vi "First.vi"(7 "Address":string, 8 "Error In":errorcluster) -> (0 "Error Out":errorcluster)   [LabVIEW 2018, in "Tests.lvlib" / "Known Hosts.lvlib"]
uses:
  Known Hosts.lvlib
  src/Toolkit/API/Known Hosts/API/Typedefs/Get Results.ctl
  <vilib>/Utility/error.llb/Clear Errors.vi
  <vilib>/Utility/file.llb/Is Path and Not Empty.vi
  <vilib>/Utility/sysdir.llb/Get System Directory.vi
  src/Toolkit/API/Known Host/Support/Create from Known Hosts.vi
  src/Toolkit/API/Known Host/Support/Destroy to Known Hosts.vi
  <vilib>/addons/_JKI Toolkits/Caraya/classes/Test/Test.lvclass
  <vilib>/addons/_JKI Toolkits/Caraya/classes/Assert/Assert.lvclass
  src/Toolkit/API/Known Hosts/Known Hosts.lvclass
  Tests.lvlib
  src/Toolkit/API/Session/Session.lvclass
  src/Toolkit/API/Known Host/Known Host.lvclass
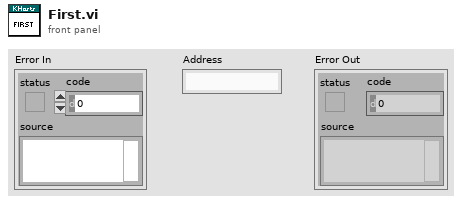
[diagram p1: front panel]
types:
  T1 = typedef "Toolkit.lvlib/Known Hosts.lvclass/Get Results.ctl" = enum32{"Success", "End of Hosts"}
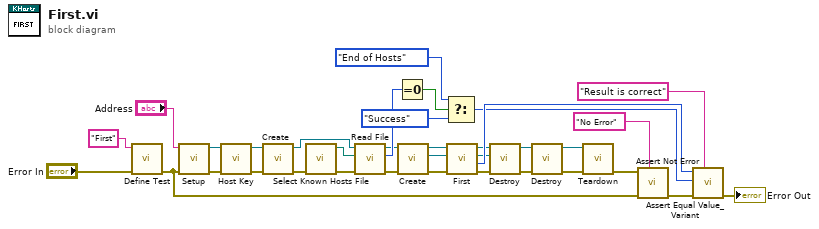
[diagram p0: block diagram]
diagram:
  n1 = call <vilib>:"Define Test.vi"("error in (no error)"="Error In", "Label (VI Title)"="First") -> ("error out"=w22:errorcluster)  [unwired: 9 in]
  n2 = call "Setup.vi"("Error In"=w22, "Address In"="Address") -> ("Error Out"=w23:errorcluster, "Sesssion"=w24:refnum<class "Session.lvclass">)  [unwired: 7 in, 1 out]
  n3 = call "Host Key.vi"("Error In"=w23, "Session In"=w24) -> ("Error Out"=w25:errorcluster, "Sesssion Out"=w20:refnum<class "Session.lvclass">)  [unwired: 6 in, 2 out]
  n4 = call "Create.vi"("Error In"=w25, "Session"=w20) -> ("Error Out"=w31:errorcluster, "Known Hosts"=w32:refnum<class "Known Hosts.lvclass">)  [unwired: 8 in]
  n5 = call "Select Known Hosts File.vi"("Error In"=w31) -> ("Error Out"=w30:errorcluster, "Known Hosts File"=w29:path)  [unwired: 9 in]
  n6 = call "Read File.vi"("Error In"=w30, "File"=w29, "KnownHosts In"=w32) -> ("Error Out"=w17:errorcluster, "Count"=w14:u64, "KnownHosts Out"=w8:refnum<class "Known Hosts.lvclass">)  [unwired: 6 in]
  n7 = Equal To 0?(x=w14) -> (x = 0?=w13:bool)
  n8 = call-poly "Create.vi"("Error In"=w17, "Known Hosts In"=w8) -> ("Error Out"=w16:errorcluster, "Known Host"=w6:refnum<class "Known Host.lvclass">, "Known Hosts Out"=w7:refnum<class "Known Hosts.lvclass">)  [unwired: 7 in]
  n9 = Select(t=Get_Results."End of Hosts" ("Get Result"), s=w13, f=Get_Results."Success" ("Get Result")) -> (s? t:f=w10:T1)
  n10 = call "First.vi"("Error In"=w16, "Known Host In"=w6, "KnownHosts In"=w7) -> ("Error Out"=w2:errorcluster, "Result"=w15:T1, "Known Host Out"=w3:refnum<class "Known Host.lvclass">, "KnownHosts Out"=w5:refnum<class "Known Hosts.lvclass">)  [unwired: 5 in]
  n11 = call-poly "Destroy.vi"("Error In"=w2, "Known Host"=w3, "KnownHosts In"=w5) -> ("Error Out"=w1:errorcluster, "KnownHosts Out"=w4:refnum<class "Known Hosts.lvclass">)  [unwired: 7 in]
  n12 = call "Destroy.vi"("Error In"=w1, "KnownHosts"=w4) -> ("Error Out"=w19:errorcluster, "Session"=w9:refnum<class "Session.lvclass">)  [unwired: 8 in]
  n13 = call "Teardown.vi"("Error In"=w19, "Session"=w9) -> ("Error Out"=w18:errorcluster)  [unwired: 9 in]
  n14 = call <vilib>:"Assert Not Error.vi"("Label"="No Error", "error in (no error)"=w22, "Not Error?"=w18) -> ("error out"=w28:errorcluster)  [unwired: 8 in]
  n15 = call <vilib>:"Assert Equal Value_Variant.vi"("Label"="Result is correct", "error in (no error)"=w28, "Y"=w10, "X"=w15) -> ("error out"=→"Error Out":errorcluster)  [unwired: 7 in]
